vi "queryEsh2.vi"() -> (3 "Array":cluster{"name":string, "params":variant[]}[](array[cluster]))   [LabVIEW 2013]
uses:
  Vireo.framework
panel:
  out "Numeric":i32
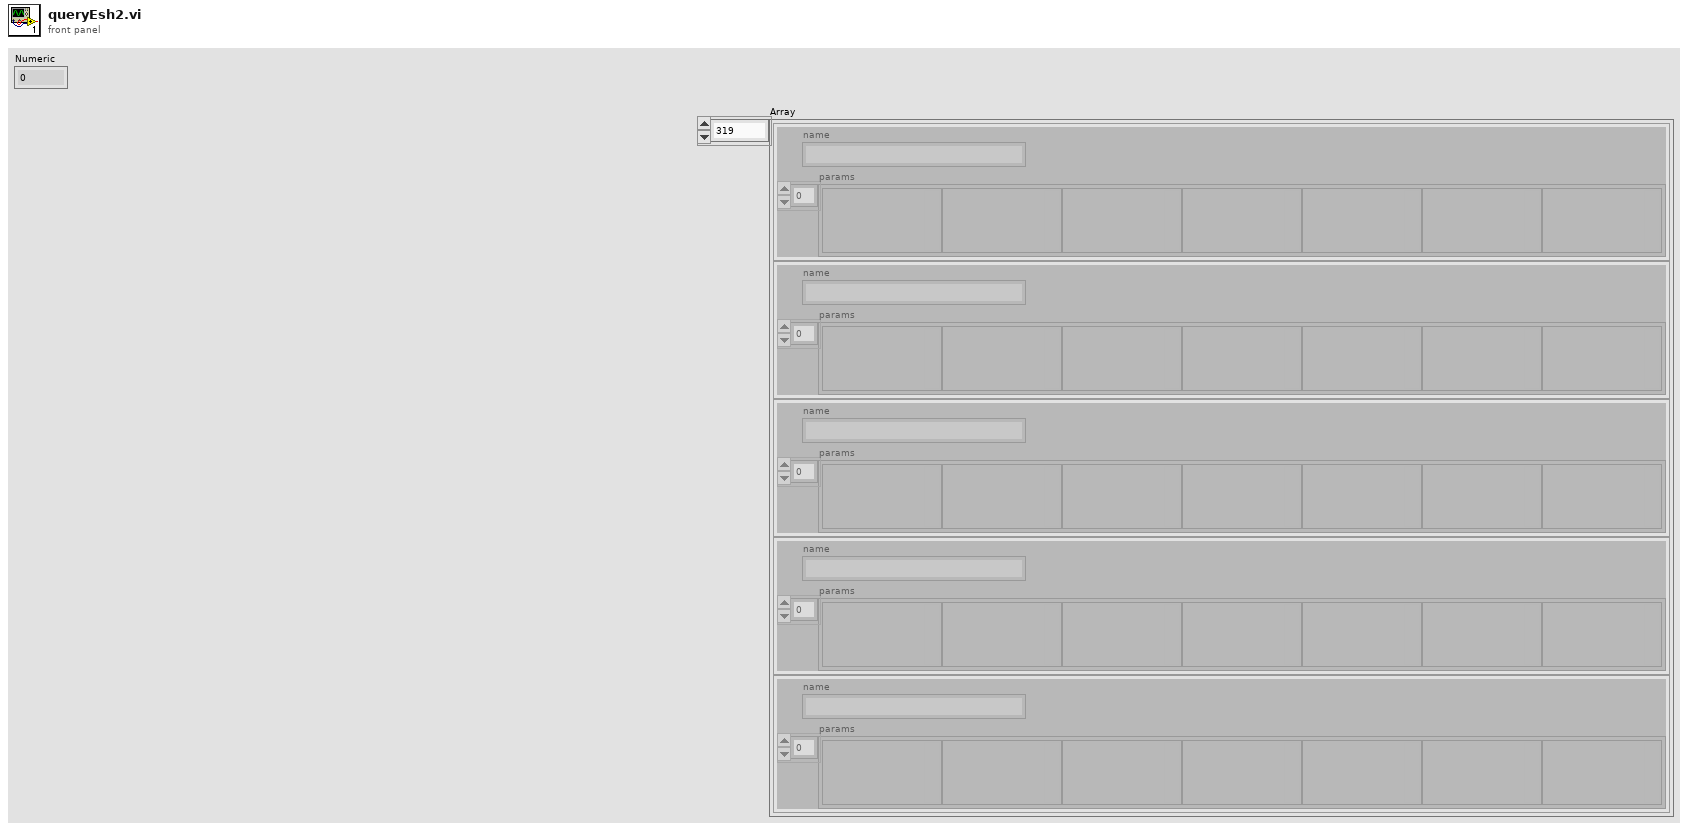
[diagram p1: front panel]
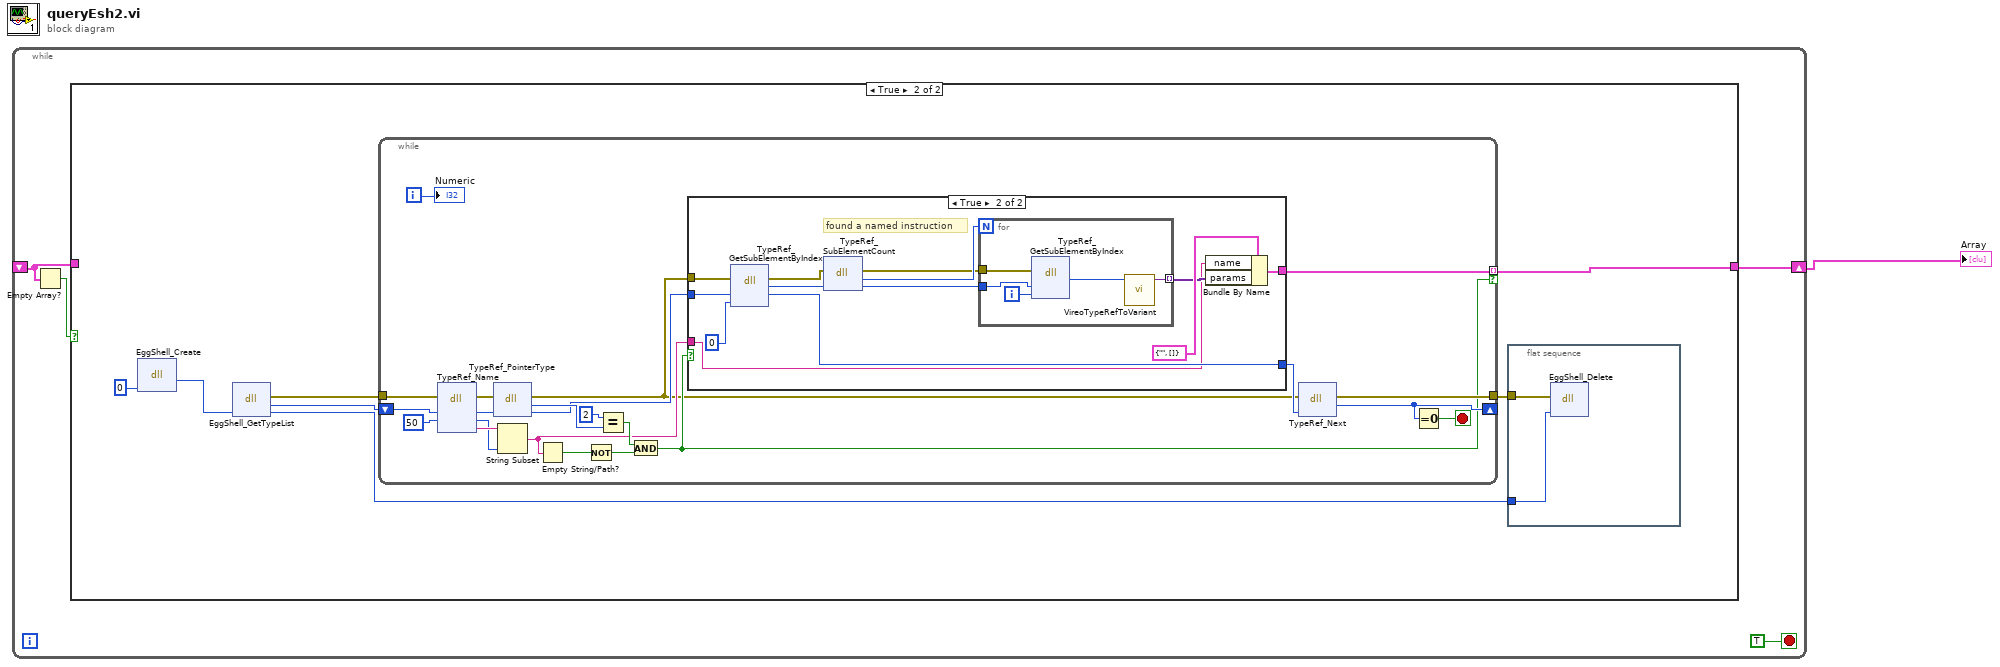
[diagram p0: block diagram]
diagram:
  n1 = while {
    shift-right: [w5] -> w1
    shift-left: _ -> [w3]
    stop <- TRUE stop-if-true
    n2 = Empty Array?(array=w3) -> (empty?=w4:bool)
    n3 = case shown="True" w4 {
      tunnel: [w6 w7] -> w5
      tunnel: w3 -> [w6 _]
      frame False {
      }
      frame True {
        n4 = dll-call lib="Macintosh HD/Users/paulaustin/repos/NI_VireoSDK/sample-vis/VireoFunctionNode/Vireo.framework" fn="EggShell_Create"("parent"=i64 0) -> ("return type"=w12:i64)  [unwired: 4 in, 2 out]
        n5 = dll-call lib="Macintosh HD/Users/paulaustin/repos/NI_VireoSDK/sample-vis/VireoFunctionNode/Vireo.framework" fn="EggShell_GetTypeList"("pShell"=w12) -> (error out=w8:errorcluster, "typeRef"=w11:i64, "pShell"=w10:i64)  [unwired: 3 in, 1 out]
        n6 = while {
          shift-right: [w33] -> _
          shift-left: w11 -> [w36]
          tunnel: [w35] -> w9
          tunnel: w8 -> [w22]
          tunnel: [w18] -> w7 mode=indexing if=w17
          i -> [w30]
          stop <- w32 stop-if-true
          n7 = dll-call lib="Macintosh HD/Users/paulaustin/repos/NI_VireoSDK/sample-vis/VireoFunctionNode/Vireo.framework" fn="TypeRef_Name" label="Name"(error in=w22, "typeRef"=w36, "bufferSize"=50) -> (error out=w23:errorcluster, "typeRef"=w29:i64, "bufferSize"=w31:i32, "name"=w34:string)  [unwired: 4 in, 1 out]
          n8 = dll-call lib="Macintosh HD/Users/paulaustin/repos/NI_VireoSDK/sample-vis/VireoFunctionNode/Vireo.framework" fn="TypeRef_PointerType" label="PointerType"(error in=w23, "typeRef"=w29) -> (error out=w16:errorcluster, "encoding"=w28:i32, "typeRef"=w20:i64)  [unwired: 2 in, 1 out]
          n9 = String Subset(string=w34, length (rest)=w31) -> (substring=w19:string)  [unwired: 1 in]
          n10 = Empty String/Path?(string/path=w19) -> (empty?=w25:bool)
          n11 = Not(x=w25) -> (.not. x?=w24:bool)
          n12 = Equal?(x=2, y=w28) -> (x = y?=w26:bool)
          n13 = And(x=w26, y=w24) -> (x .and. y?=w17:bool)
          n14 = case shown="True" w17 {
            tunnel: [w38 w49] -> w21
            tunnel: w20 -> [w38 w51]
            tunnel: w16 -> [_ w48]
            tunnel: [_ w42] -> w18
            tunnel: w19 -> [_ w41]
            frame False {
            }
            frame True {
              # "found a named instruction"
              n15 = dll-call lib="Macintosh HD/Users/paulaustin/repos/NI_VireoSDK/sample-vis/VireoFunctionNode/Vireo.framework" fn="TypeRef_GetSubElementByIndex" label="GetSubElement"(error in=w48, "typeRef"=w51, "index"=0) -> (error out=w40:errorcluster, "typeRef"=w47:i64, "typeRef"=w49:i64)  [unwired: 3 in, 1 out]
              n16 = dll-call lib="Macintosh HD/Users/paulaustin/repos/NI_VireoSDK/sample-vis/VireoFunctionNode/Vireo.framework" fn="TypeRef_SubElementCount" label="GetSubElementCount"(error in=w40, "typeRef"=w47) -> (error out=w39:errorcluster, "count"=w46:i32, "typeRef"=w45:i64)  [unwired: 2 in, 1 out]
              n17 = for {
                N: w46 -> [_]
                tunnel: w45 -> [w56]
                tunnel: [w52] -> w43 mode=indexing
                tunnel: w39 -> [w54]
                i -> [w55]
                n18 = dll-call lib="Macintosh HD/Users/paulaustin/repos/NI_VireoSDK/sample-vis/VireoFunctionNode/Vireo.framework" fn="TypeRef_GetSubElementByIndex" label="GetSubElement"(error in=w54, "typeRef"=w56, "index"=w55) -> ("typeRef"=w53:i64)  [unwired: 4 in, 2 out]
                n19 = call "VireoTypeRefToVariant.vi"("typeRef"=w53) -> ("variant"=w52:variant)  [unwired: 10 in]
              }
              n20 = Bundle By Name(cluster=cluster{"name":string, "params":variant[]} {"name"="", "params"=[]}, "name"=w41, "params"=w43) -> (w42:cluster{"name":string, "params":variant[]})
            }
          }
          n21 = dll-call lib="Macintosh HD/Users/paulaustin/repos/NI_VireoSDK/sample-vis/VireoFunctionNode/Vireo.framework" fn="TypeRef_Next"(error in=w16, "typeRef"=w21) -> (error out=w35:errorcluster, "typeRef"=w33:i64)  [unwired: 3 in, 1 out]
          n22 = Equal To 0?(x=w33) -> (x = 0?=w32:bool)
          "Numeric" <- w30
        }
        n23 = flat-sequence {
          tunnel: w10 -> [w15]
          tunnel: w9 -> [w14]
          frame #0 {
            n24 = dll-call lib="Macintosh HD/Users/paulaustin/repos/NI_VireoSDK/sample-vis/VireoFunctionNode/Vireo.framework" fn="EggShell_Delete"(error in=w14, "shell"=w15) -> ()  [unwired: 4 in, 2 out]
          }
        }
      }
    }
  }
  "Array" <- w1
